vi "Each_Data_struct_Add.vi"(1 "Active Sensors":bool[](array[boolean]), 2 "chk2scan":bool, 5 "Controls[]":refnum<vi>[](array[refnum]), 7 "Data_struct输入":refnum<k24>[](array[refnum]), 11 "错误输入（无错误）":errorcluster, 12 "sweep_count":i32, 13 "Meas_rang":i32[](array[numeric])) -> (6 "Data_struct输出":refnum<k24>[](array[refnum]), 15 "错误输出":errorcluster)   [LabVIEW 2017]
doc: "for measurement power data"
uses:
  D:/test/PDLSTS/LV_PDL LvVer17.0/LV_PDL_x64/DLL/STSProcess.dll
  DLL/STSProcess.dll
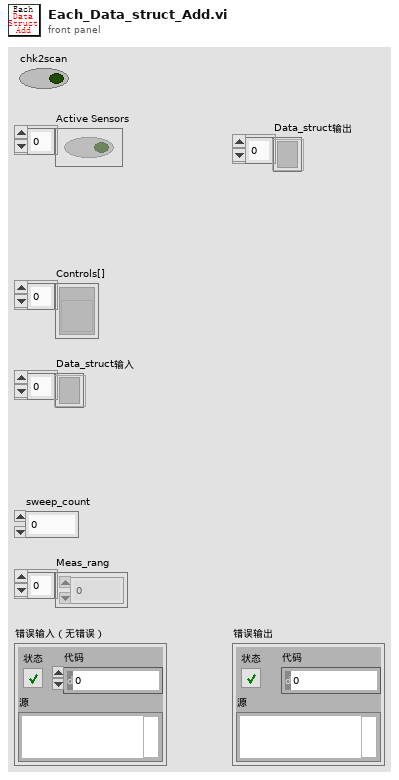
[diagram p1: front panel]
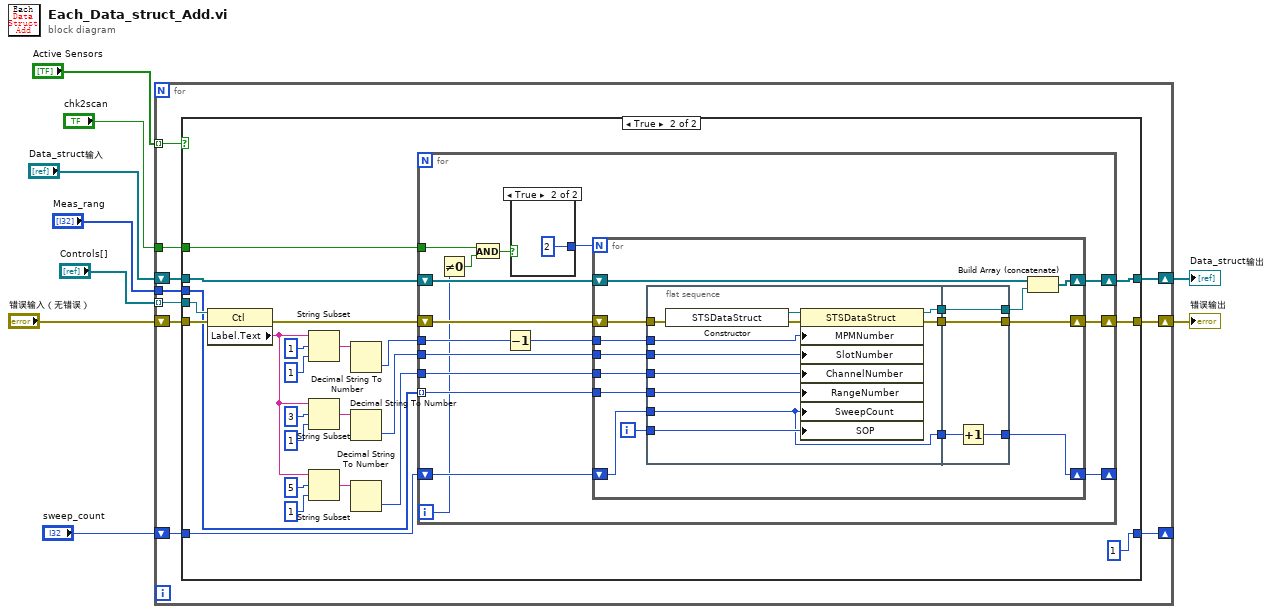
[diagram p0: block diagram]
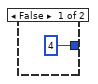
[diagram p3: hidden frame]
diagram:
  n1 = for {
    tunnel: "Active Sensors" -> [w19] mode=indexing
    tunnel: "Controls[]" -> [w18] mode=indexing
    tunnel: "Meas_rang" -> [w17]
    shift-right: [w15] -> w1
    shift-left: "Data_struct输入" -> [w16]
    shift-right: [w14] -> w2
    shift-left: "错误输入（无错误）" -> [w13]
    tunnel: "chk2scan" -> [w11]
    shift-right: [w10] -> _
    shift-left: "sweep_count" -> [w12]
    n2 = case shown="True" w19 {
      tunnel: w18 -> [_ w45]
      tunnel: w16 -> [w22 w27]
      tunnel: [w22 w33] -> w15
      tunnel: [w21 w30] -> w14
      tunnel: w13 -> [w21 w29]
      tunnel: w17 -> [_ w28]
      tunnel: w12 -> [w20 w25]
      tunnel: w11 -> [_ w24]
      tunnel: [w20 1] -> w10
      frame False {
      }
      frame True {
        n3 = property class="Ctl"(reference=w45, error in=w29) -> (error out=w26:errorcluster, "Label.Text"=w40:string)  [unwired: 1 out]
        n4 = String Subset(string=w40, offset (0)=1 ("偏移量(0)"), length (rest)=1 ("长度（剩余）")) -> (substring=w36:string)
        n5 = String Subset(string=w40, offset (0)=3 ("偏移量(0)"), length (rest)=1 ("长度（剩余）")) -> (substring=w37:string)
        n6 = String Subset(string=w40, offset (0)=5 ("偏移量(0)"), length (rest)=1 ("长度（剩余）")) -> (substring=w35:string)
        n7 = Decimal String To Number(string=w36) -> (number=w34:i32)  [unwired: 2 in, 1 out]
        n8 = Decimal String To Number(string=w37) -> (number=w32:i32)  [unwired: 2 in, 1 out]
        n9 = Decimal String To Number(string=w35) -> (number=w31:i32)  [unwired: 2 in, 1 out]
        n10 = for {
          tunnel: w34 -> [w61]
          tunnel: w32 -> [w59]
          tunnel: w31 -> [w58]
          tunnel: w28 -> [w55] mode=indexing
          shift-right: [w56] -> w30
          shift-left: w26 -> [w50]
          shift-right: [w60] -> w33
          shift-left: w27 -> [w51]
          tunnel: w24 -> [w48]
          shift-right: [w47] -> _
          shift-left: w25 -> [w49]
          i -> [w46]
          n11 = Not Equal To 0?(x=w46) -> (x != 0?=w54:bool)
          n12 = And(x=w48, y=w54) -> (x .and. y?=w53:bool)
          n13 = Decrement(x=w61) -> (x-1=w57:i32)
          n14 = case shown="True" w53 {
            tunnel: [4 2] -> w52
            frame False {
            }
            frame True {
            }
          }
          n15 = for {
            N: w52 -> [_]
            tunnel: w59 -> [w73]
            tunnel: w58 -> [w72]
            tunnel: w57 -> [w71]
            tunnel: w55 -> [w69]
            shift-right: [w70] -> w56
            shift-left: w50 -> [w65]
            shift-right: [w74] -> w60
            shift-left: w51 -> [w76]
            shift-right: [w62] -> w47
            shift-left: w49 -> [w64]
            i -> [w68]
            n16 = flat-sequence {
              tunnel: w73 -> [w84]
              tunnel: w72 -> [w83]
              tunnel: w71 -> [w79]
              tunnel: w69 -> [w81]
              tunnel: w68 -> [w78]
              tunnel: [w85] -> w67
              tunnel: [w82] -> w66
              tunnel: w65 -> [w80]
              tunnel: w64 -> [w77]
              tunnel: [w77] -> w63
              tunnel: [w90] -> w70
              tunnel: [w91] -> w75
              tunnel: w67 -> [w91]
              tunnel: w66 -> [w90]
              tunnel: w63 -> [w89]
              tunnel: [w88] -> w62
              frame #0 {
                n17 = constructor class="STSDataStruct"(error in=w80) -> (reference out=w87:refnum<k24>, error out=w86:errorcluster)  [unwired: 2 in, 1 out]
                n18 = property on="属性节点" class="STSDataStruct"(reference=w87, error in=w86, "MPMNumber"=w79, "SlotNumber"=w84, "ChannelNumber"=w83, "RangeNumber"=w81, "SweepCount"=w77, "SOP"=w78) -> (reference out=w85:refnum<k24>, error out=w82:errorcluster)
              }
              frame #1 {
                n19 = Increment(x=w89) -> (x+1=w88:i32)
              }
            }
            n20 = Build Array (concatenate)(w76, w75) -> (w74:refnum<k24>[])
          }
        }
      }
    }
  }
  "错误输出" <- w2
  "Data_struct输出" <- w1
